vi "Read OOB DVR.vi"(8 "error in":errorcluster, 11 "OOB in":refnum<class "CIFOutOfBand.lvclass">) -> (0 "error out":errorcluster, 1 "New Commands":bool, 2 "Commands (bitwise)":u64, 3 "OOB out":refnum<class "CIFOutOfBand.lvclass">)   [LabVIEW 2021, in "CIFOutOfBand.lvclass"]
uses:
  CIFOutOfBand.lvclass
  CIFOutOfBand.lvclass/CIFOutOfBand.ctl
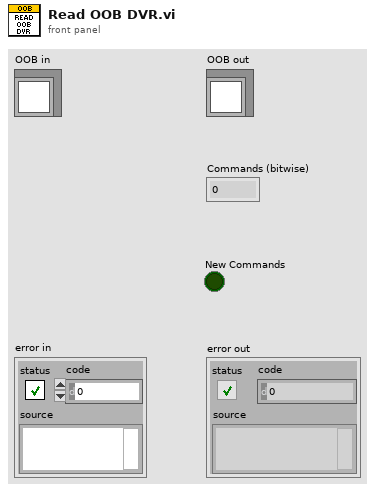
[diagram p1: front panel]
types:
  T1 = typedef "CIFOutOfBand2.lvclass/OOB Container.ctl" = cluster{"Commands":u64, "Payload":variant}
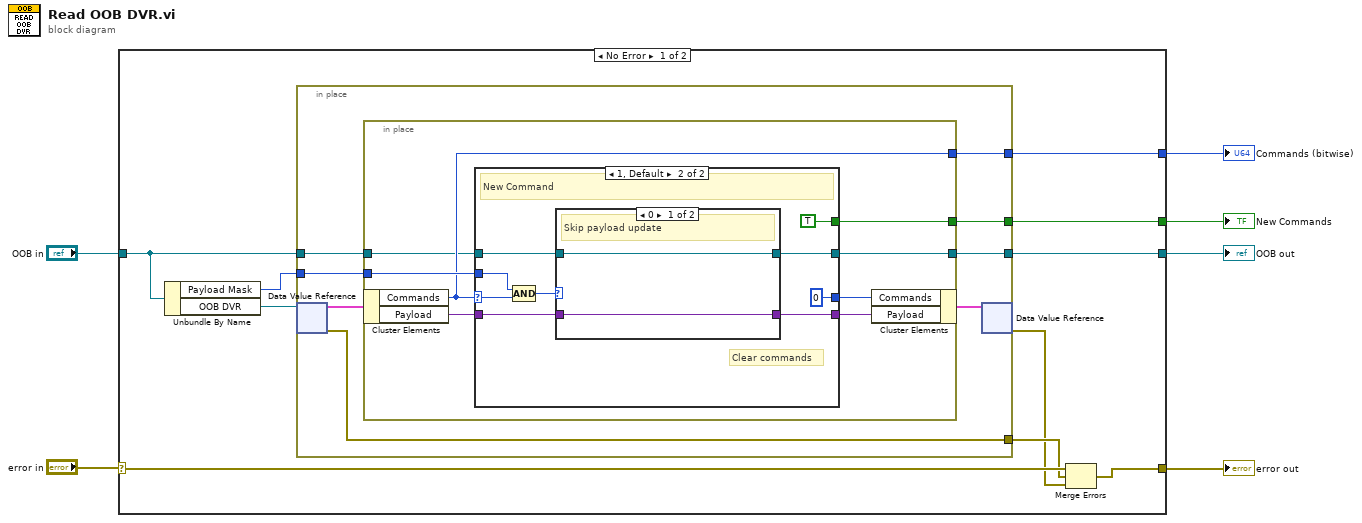
[diagram p0: block diagram]
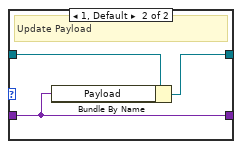
[diagram p3: hidden frame]
diagram:
  n1 = case shown="No Error" "error in" {
    selector: "error in" -> [w15 w51]
    tunnel: [w16 w51] -> w5
    tunnel: "OOB in" -> [w8 w50]
    tunnel: [w7 w50] -> w3
    tunnel: [w14 _] -> w2
    tunnel: [w13 _] -> w1
    frame No Error {
      n2 = Unbundle By Name(w8) -> ("Payload Mask"=w9:u64, "OOB DVR"=w12:refnum<data-value>)
      n3 = in-place {
        in-place-border: [w24] -> w11
        in-place-border: w9 -> [w21]
        in-place-border: [w20] -> w14
        in-place-border: [w19] -> w13
        in-place-border: w8 -> [w18]
        in-place-border: [w17] -> w7
        n4 = in-place-dvr #1(w12) -> (w23:T1, w24:errorcluster)
        n5 = in-place {
          in-place-border: w21 -> [w29]
          in-place-border: [w28] -> w20
          in-place-border: [w27] -> w19
          in-place-border: w18 -> [w26]
          in-place-border: [w25] -> w17
          n6 = in-place-cluster #2(w23) -> ("Commands"=w27:u64, "Payload"=w32:variant)
          n7 = case shown="1, Default" w27 {
            selector: w27 -> [w34 w42]
            tunnel: w32 -> [w35 w43]
            tunnel: [w35 w41] -> w31
            tunnel: [w34 u64 0 ("Commands")] -> w30
            tunnel: w29 -> [_ w39]
            tunnel: [_ TRUE] -> w28
            tunnel: w26 -> [w33 w37]
            tunnel: [w33 w36] -> w25
            frame 0 {
              # "No new command"
            }
            frame 1, Default {
              # "Clear commands"
              # "New Command"
              n8 = Compound Arithmetic op=AND(w39, w42) -> (w44:u64)
              n9 = case shown="0" w44 {
                tunnel: w43 -> [w46 w48]
                tunnel: [w46 w48] -> w41
                tunnel: w37 -> [w45 w49]
                tunnel: [w45 w47] -> w36
                frame 0 {
                  # "Skip payload update"
                }
                frame 1, Default {
                  # "Update Payload"
                  n10 = Bundle By Name(cluster=w49, "Payload"=w48) -> (w47:refnum<class "CIFOutOfBand.lvclass">)
                }
              }
            }
          }
          n11 = in-place-cluster #2("Commands"=w30, "Payload"=w31) -> (w22:T1)
        }
        n12 = in-place-dvr #1(w22) -> (w10:errorcluster)  [unwired: 1 out]
      }
      n13 = Merge Errors(w15, w11, w10) -> (w16:errorcluster)
    }
    frame Error {
    }
  }
  "error out" <- w5
  "OOB out" <- w3
  "New Commands" <- w2
  "Commands (bitwise)" <- w1
